vi "input condition.vi"() -> (0 "input Parameter 2":T1, 3 "input envTemp. & elecFee 2":cluster{"Temp.":dbl[], "elecFee":dbl[]})   [LabVIEW 2014]
panel:
  in  "url":string="https://e-service.cwb.gov.tw/HistoryDataQuery/index.jsp"
  in  "WebBrowser":refnum<k7>(container)
  in  "input Parameter":T1={"input COP of ACs"=3.0, "input setDay Temp"=22.0, "input setNight Temp."=20.0}
  in  "input envTemp. & elecFee":cluster{"Temp.":dbl[], "elecFee":dbl[]}={"Temp."=[29.6, 26.5, 26.8, 26.8, 26.5, 26.9, 27.8, 28.5, 26.3, 30.1, 33.3, 33.4, 33.9, 32.2, 32.7, 32.7, 32.4, 31.5, 30.5, 29.7, 28.3, 28.2, 27.9, 27.5], "elecFee"=[2.2, 2.2, 2.2, 2.2, 2.2, 2.2, 2.2, 2.2, 3.5, 3.5, 3.5, 3.5, 3.5, 3.5, 3.5, 3.5, 3.5, 3.5, 3.5, 3.5, 3.5, 3.5, 2.2, 2.2]}
  in  "OK Button":bool
  # "0~1"
  # "1~2"
  # "2~3"
  # "3~4"
  # "4~5"
  # "5~6"
  # "6~7"
  # "7~8"
  # "8~98~9"
  # "9~10"
  # "10~11"
  # "11~12"
  # "12~13"
  # "13~14"
  # "14~15"
  # "15~16"
  # "16~17"
  # "17~18"
  # "18~19"
  # "19~20"
  # "21~21"
  # "21~22"
  # "22~23"
  # "23~24"
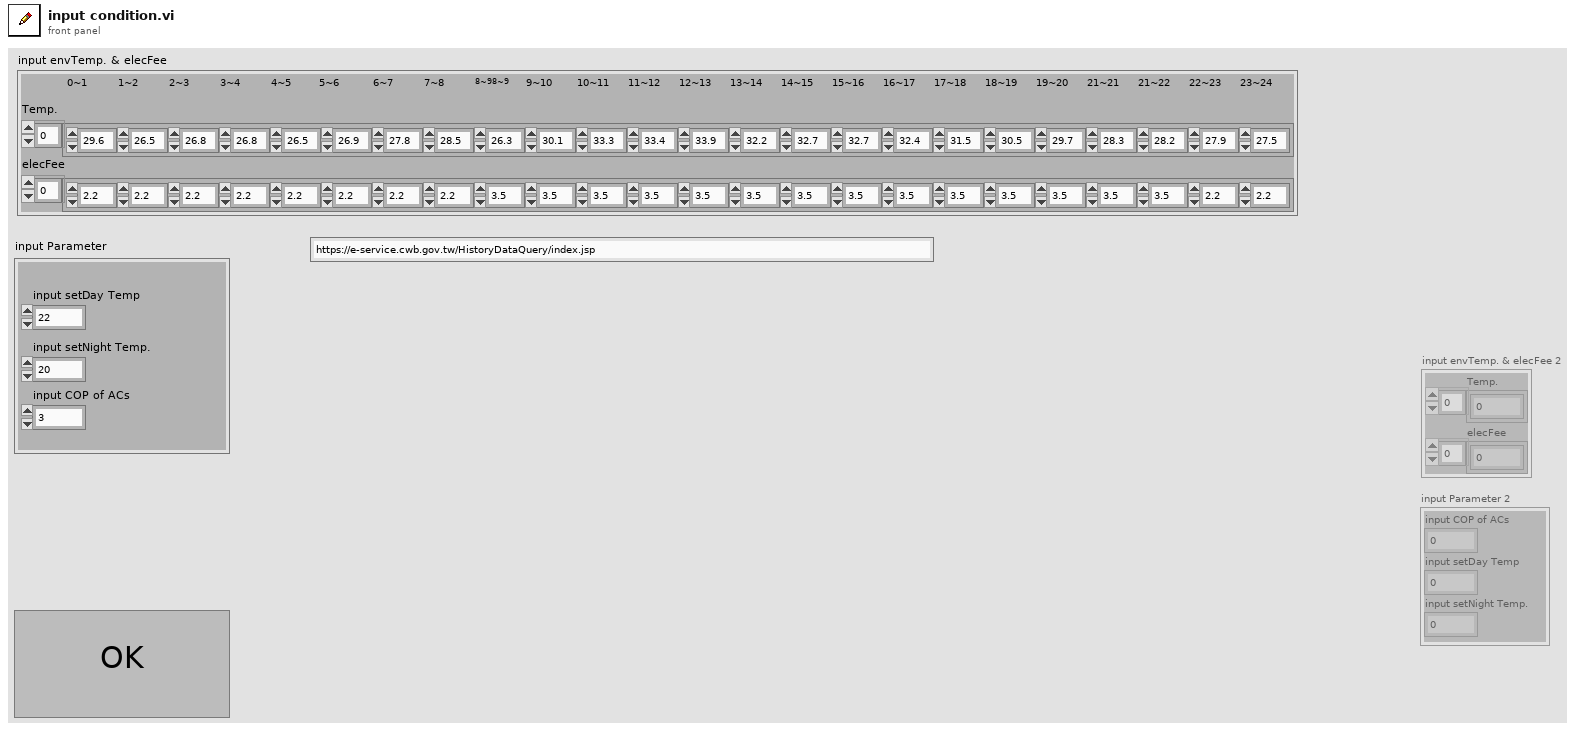
[diagram p1: front panel]
types:
  T1 = cluster{"input COP of ACs":dbl, "input setDay Temp":dbl, "input setNight Temp.":dbl}
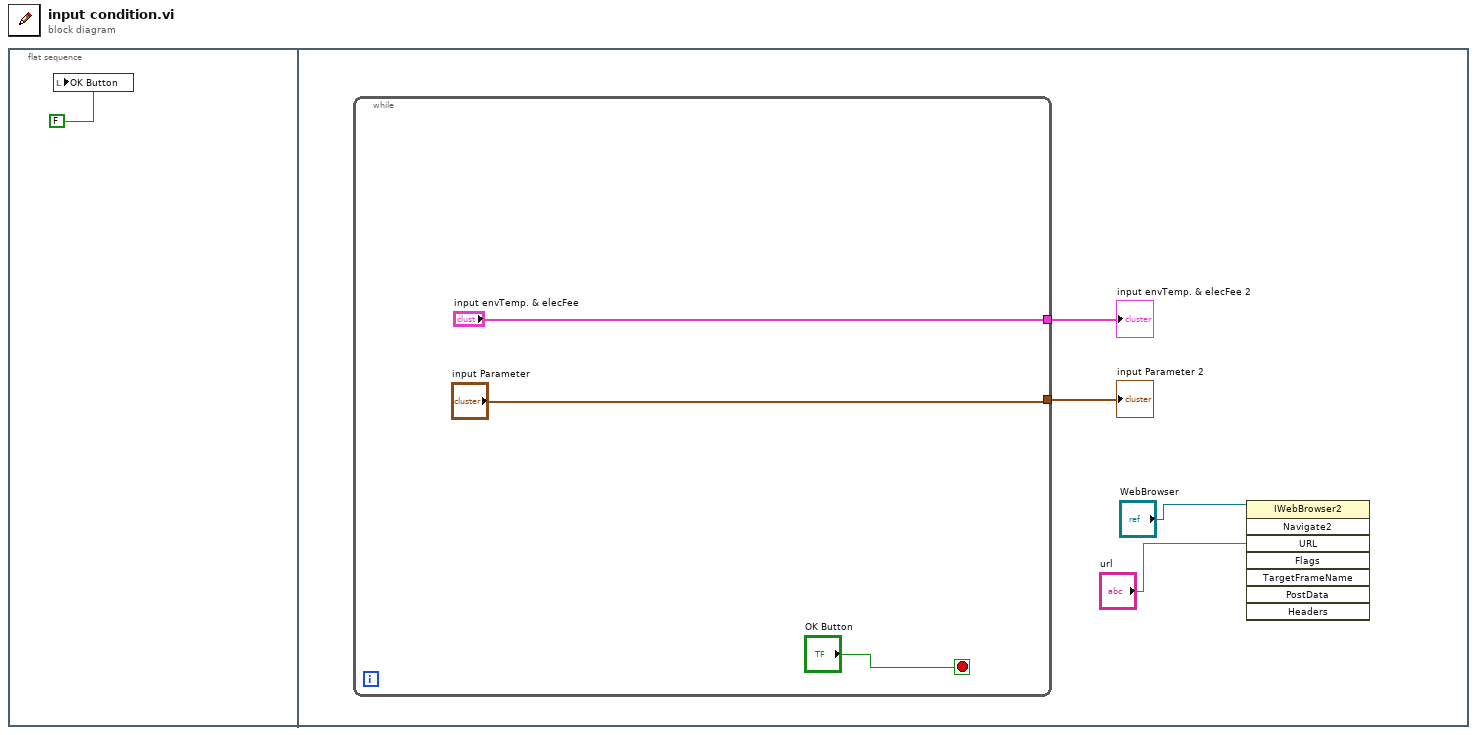
[diagram p0: block diagram]
diagram:
  n1 = flat-sequence {
    frame #0 {
      n2 = local write "OK Button"(FALSE) -> ()
    }
    frame #1 {
      n3 = while {
        tunnel: ["input envTemp. & elecFee"] -> w5
        tunnel: ["input Parameter"] -> w4
        stop <- "OK Button" stop-if-true
      }
      "input envTemp. & elecFee 2" <- w5
      "input Parameter 2" <- w4
      n4 = invoke class="IWebBrowser2" method="Navigate2"(reference="WebBrowser", "URL"="url") -> ()  [unwired: 6 in, 8 out]
    }
  }
